vi "Variable@LSetIndexValue__Parameter.vi"(1 "ParamterIn":string) -> (0 "ParamterOut":string)   [LabVIEW 2019]
panel:
  in  "Index":string(combo)
  in  "Section":string(combo)
  in  "Value":string(combo)
  in  "ParameterName":string(combo)
  in  "Confirm":bool
  # "Variable@LSetIndexValue $Variable,$Index,$Value(,$Section)"
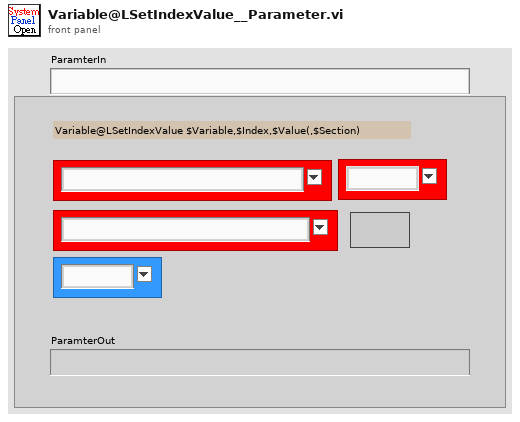
[diagram p1: front panel]
types:
  T1 = enum16{"Get", "Init", "Set", "Delete", "GetElement", "Inc", "Dec", "ReName"}
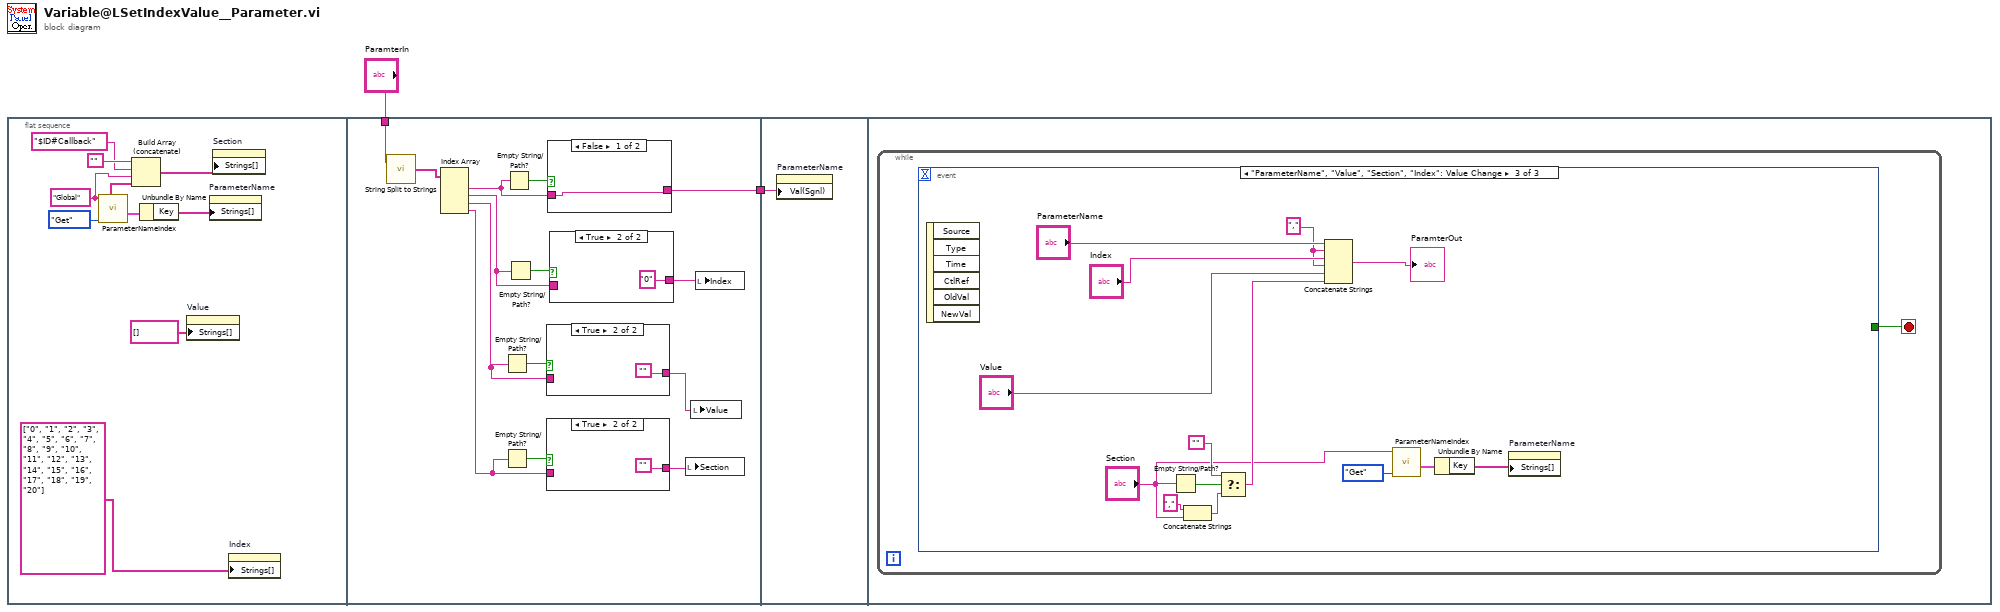
[diagram p0: block diagram]
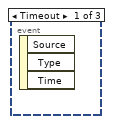
[diagram p6: hidden frame]
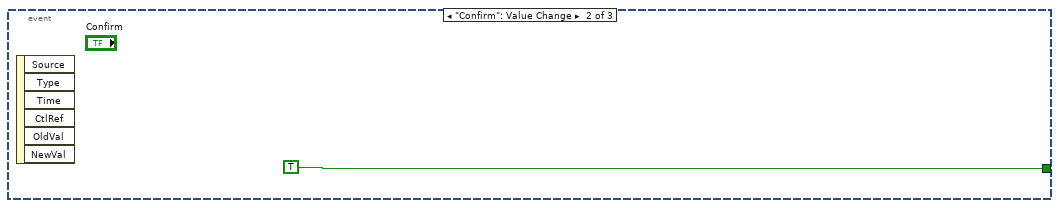
[diagram p7: hidden frame]
diagram:
  n1 = flat-sequence {
    tunnel: "ParamterIn" -> [w22]
    tunnel: [w24] -> w1
    tunnel: w1 -> [w35]
    frame #0 {
      w5 = "Global" ("VariableSection")
      n2 = call "ParameterNameIndex.vi"("OP"=T1."Get", "VariableSection"=w5) -> ("GlobalKeyValue"=w12:cluster{"Key":string[], "Value":string[]}, "SectionList"=w6:string[])  [unwired: 3 in, 5 out]
      n3 = Build Array (concatenate)("", "$ID#Callback" ("VariableSection"), w5, w6) -> (w4:string[])
      n4 = Unbundle By Name(w12) -> ("Key"=w11:string[])
      n5 = property on="Value" class="CmbBox"("Strings[]"=string[] [] ("Strings []")) -> ()  [unwired: 2 in, 2 out]
      n6 = property on="ParameterName" class="CmbBox"("Strings[]"=w11) -> ()  [unwired: 2 in, 2 out]
      n7 = property on="Section" class="CmbBox"("Strings[]"=w4) -> ()  [unwired: 2 in, 2 out]
      n8 = property on="Index" class="CmbBox"("Strings[]"=string[] ["0", "1", "2", "3", "4", "5", "6", "7", "8", "9", "10", "11", "12", "13", "14", "15", "16", "17", "18", "19", "20"] ("Strings []")) -> ()  [unwired: 2 in, 2 out]
    }
    frame #1 {
      n9 = call "String Split to Strings.vi"("String"=w22) -> ("Array"=w21:string[])  [unwired: 1 in]
      n10 = Index Array(array=w21) -> (element #1=w20:string, element #2=w14:string, element #3=w16:string, element #4=w17:string)  [unwired: 4 in]
      n11 = Empty String/Path?(string/path=w16) -> (empty?=w25:bool)
      n12 = Empty String/Path?(string/path=w17) -> (empty?=w19:bool)
      n13 = Empty String/Path?(string/path=w20) -> (empty?=w26:bool)
      n14 = Empty String/Path?(string/path=w14) -> (empty?=w15:bool)
      n15 = case shown="True" w25 {
        tunnel: w16 -> [w31 _]
        tunnel: [w31 ""] -> w23
        frame False {
        }
        frame True {
        }
      }
      n16 = case shown="True" w19 {
        tunnel: w17 -> [w29 _]
        tunnel: [w29 ""] -> w18
        frame False {
        }
        frame True {
        }
      }
      n17 = case shown="False" w26 {
        tunnel: w20 -> [w33 w34]
        tunnel: [w33 w34] -> w24
        frame False {
        }
        frame True {
        }
      }
      n18 = case shown="True" w15 {
        tunnel: w14 -> [w27 _]
        tunnel: [w27 "0"] -> w13
        frame False {
        }
        frame True {
        }
      }
      n19 = local write "Section"(w18) -> ()
      n20 = local write "Value"(w23) -> ()
      n21 = local write "Index"(w13) -> ()
    }
    frame #2 {
      n22 = property on="ParameterName" class="CmbBox"("Val(Sgnl)"=w35) -> ()  [unwired: 2 in, 2 out]
    }
    frame #3 {
      n23 = while {
        stop <- w36 stop-if-true
        n24 = event shown="[2] \"ParameterName\", \"Value\", \"Section\", \"Index\": Value Change" {
          selector: _ -> [_ _ _]
          dyn-events: _ -> [_ _ _]
          timeout: _ -> [_ _ _]
          tunnel: [_ TRUE _] -> w36
          event Timeout {
            n25 = event-data() -> ()  [unwired: 1 in, 3 out]
          }
          event "Confirm": Value Change {
            n26 = event-data() -> ()  [unwired: 1 in, 6 out]
          }
          event "ParameterName", "Value", "Section", "Index": Value Change {
            w43 = "," ("string")
            n27 = event-data() -> ()  [unwired: 1 in, 6 out]
            n28 = Empty String/Path?(string/path="Section") -> (empty?=w47:bool)
            n29 = Concatenate Strings("," ("string"), "Section") -> (w48:string)
            n30 = Select(t="", s=w47, f=w48) -> (s? t:f=w41:string)
            n31 = Concatenate Strings("ParameterName", w43, "Index", w43, "Value", w41) -> (→"ParamterOut":string)
            n32 = call "ParameterNameIndex.vi"("OP"=T1."Get", "VariableSection"="Section") -> ("GlobalKeyValue"=w39:cluster{"Key":string[], "Value":string[]})  [unwired: 3 in, 6 out]
            n33 = Unbundle By Name(w39) -> ("Key"=w46:string[])
            n34 = property on="ParameterName" class="CmbBox"("Strings[]"=w46) -> ()  [unwired: 2 in, 2 out]
          }
        }
      }
    }
  }
